vi "SR830 sweep tw.vi"(5 "Sweep":bool, 6 "Lock in parameters":T1={"Phase (deg)"=82.0, "TC"=7, "TC Multiplier"=5.0} {"TC Multiplier" min=0.0 max=10.0 step=1.0 format="%.2f"; "TC" items=["10 µs", "30 µs", "100 µs", "300 µs", "1 ms", "3 ms", "10 ms", "30 ms", "100 ms", "300 ms", "1 s", "3 s", "10 s", "30 s", "100 s", "300 s", "1 ks", "3 ks", "10 ks", "30 ks"]; "Phase (deg)" format="%.3f"}, 7 "Sweep frequency":T2={"Start Freq. (Hz)"=1040.0, "Stop Freq. (Hz)"=1200.0, "# of Steps"=100} {"Stop Freq. (Hz)" min=0.0 max=3000.0 step=0.001 format="%.3f"; "Start Freq. (Hz)" min=0.0 max=3000.0 step=0.001 format="%.3f"}, 8 "Lock-in GPIB address":string="0:9", 9 "SRS DS345 GPIB address":string="0:19") -> (0 "Fitting status":errorcluster[](array[cluster]), 1 "Best Fit Coefficients":dbl[][](array[numeric]) format="%#_6p", 2 "Sweep fit data":dbl[][](array[numeric]) format="%#_6p", 3 "Sweep data":dbl[][](array[numeric]) format="%#_6p")   [LabVIEW 2015]
uses:
  <vilib>/Analysis/1siggen.llb/Ramp Pattern by Samples.vi
  <vilib>/Analysis/baseanly.llb/Mean (DBL).vi
  <vilib>/gmath/NumericalOptimization/Nonlinear Curve Fit LM formula string.vi
  <vilib>/gmath/NI_Gmath.lvlib
  <vilib>/Analysis/NI_AALBase.lvlib
panel:
  out "Sweep Fit Chart":dbl[][](graph)
  out "Sweep Chart":cluster{"[0]":dbl, "[1]":dbl}(graph)
  in  "Lock-in GPIB address  (Fake)":string="1:8"
  # "width              center freq.        phase            amplitude        linear bkgd         cont bkgd\n        (Hz)                    (Hz)                (deg.)                (A)                   (A)                     (A)"
  # "X"
  # "Y"
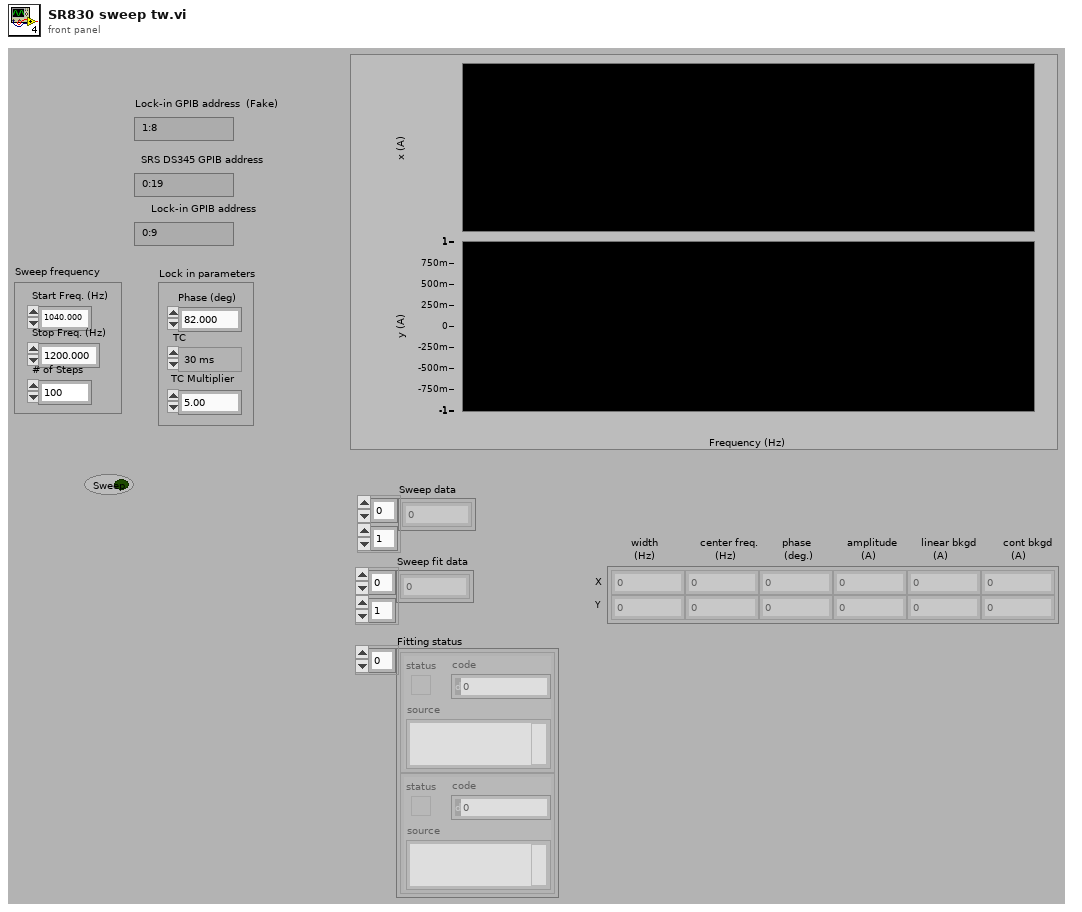
[diagram p1: front panel]
types:
  T1 = cluster{"Phase (deg)":dbl, "TC":i32, "TC Multiplier":dbl}
  T2 = cluster{"Start Freq. (Hz)":dbl, "Stop Freq. (Hz)":dbl, "# of Steps":u16}
  T3 = cluster{"Lock-in GPIB address  (Fake)":string, "Lock-in GPIB address  ":string, "SRS DS345 GPIB address":string}
  T4 = cluster{"model":string, "Parameters":string[], "x":string}
  T5 = cluster{"[0]":dbl, "[1]":dbl, "[2]":dbl, "[3]":dbl, "[4]":dbl, "[5]":dbl, "[6]":dbl, "[7]":dbl, "[8]":dbl}
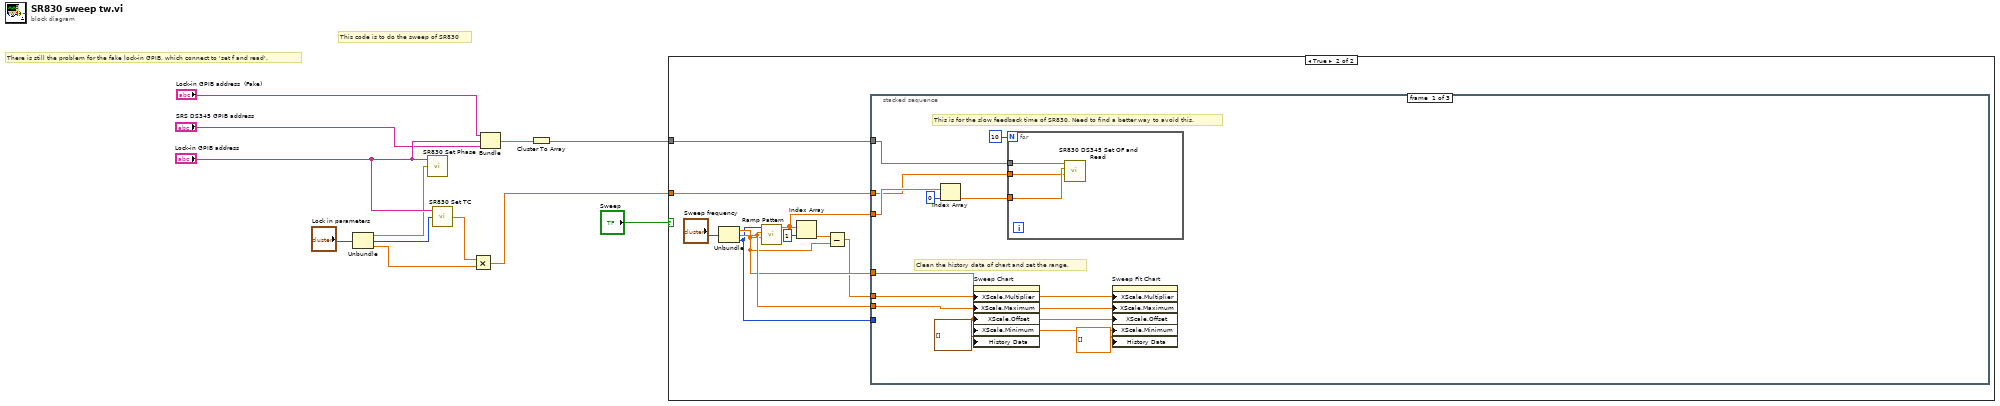
[diagram p0: block diagram]
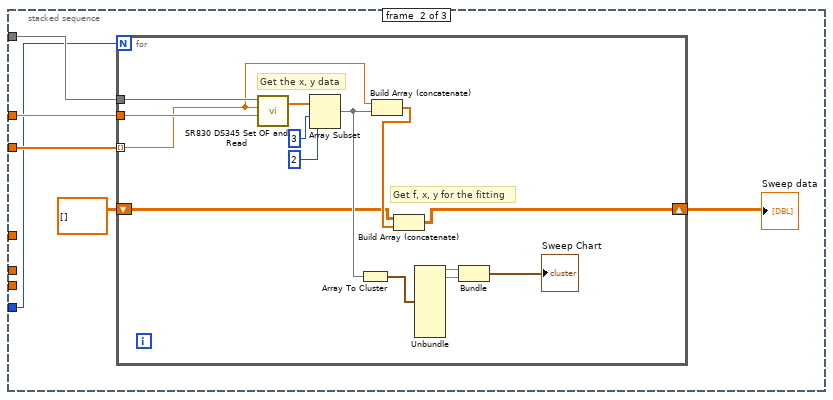
[diagram p3: hidden frame]
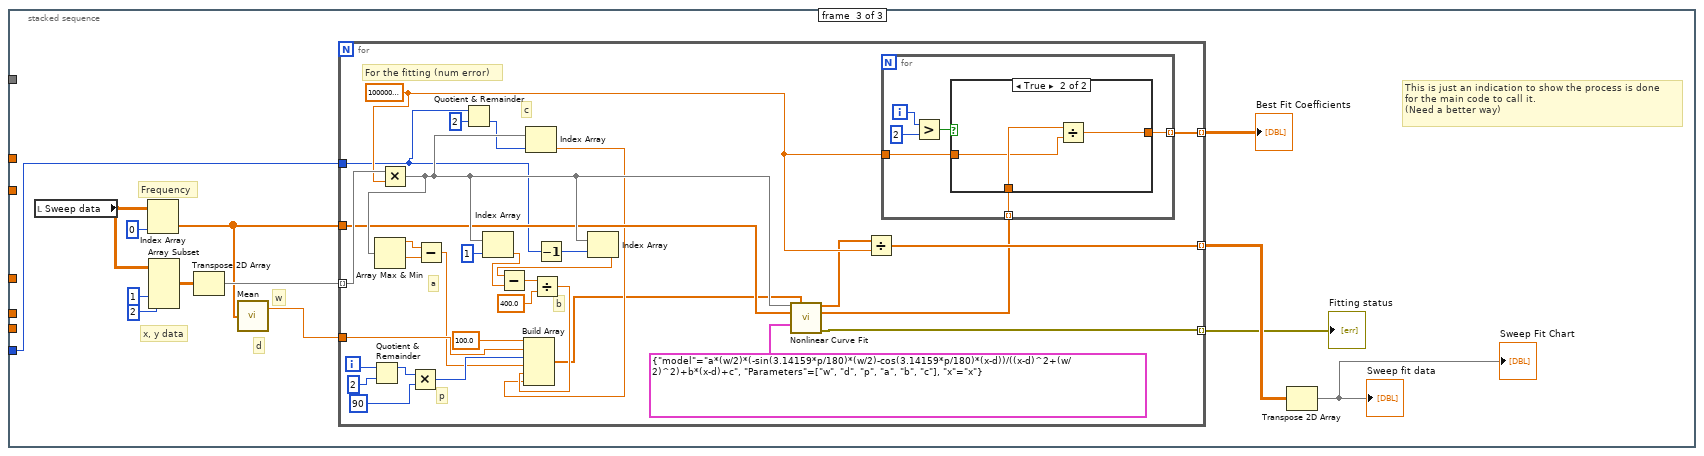
[diagram p4: hidden frame]
diagram:
  # "This code is to do the sweep of SR830"
  # "There is still the problem for the fake lock-in GPIB, which connect to 'set f and read'."
  n1 = Unbundle("Lock in parameters") -> ("Phase (deg)"=w4:dbl, "TC"=w3:i32, "TC Multiplier"=w2:dbl)
  n2 = call "SR830 Set Phase.vi"("Phase (deg)"=w4, "GPIB address"="Lock-in GPIB address") -> ()  [unwired: 2 in, 2 out]
  n3 = call "SR830 Set TC.vi"("time constant\n(10 µs : 0)"=w3, "GPIB address"="Lock-in GPIB address") -> ("tc (sec)"=w7:dbl)  [unwired: 1 in, 2 out]
  n4 = Multiply(x=w7, y=w2) -> (x*y=w6:dbl)
  n5 = Bundle("Lock-in GPIB address  (Fake)"="Lock-in GPIB address  (Fake)", "Lock-in GPIB address"="Lock-in GPIB address", "SRS DS345 GPIB address"="SRS DS345 GPIB address") -> (w9:T3)  [unwired: 1 out]
  n6 = Cluster To Array(cluster=w9) -> (array=w8:string[])
  n7 = case shown="True" "Sweep" {
    tunnel: w8 -> [_ w22]
    tunnel: w6 -> [_ w13]
    frame False {
    }
    frame True {
      n8 = Unbundle("Sweep frequency") -> ("Start Freq. (Hz)"=w17:dbl, "Stop Freq. (Hz)"=w20:dbl, "# of Steps"=w15:u16)
      n9 = call-poly <vilib>:"Ramp Pattern.vi"("start"=w17, "end"=w20, "samples"=w15) -> ("Ramp Pattern"=w14:dbl[])  [unwired: 7 in, 1 out]
      n10 = Index Array(array=w14, index=1) -> (element=w18:dbl)
      n11 = Subtract(x=w18, y=w17) -> (x-y=w16:dbl)
      n12 = stacked-sequence {
        tunnel: w22 -> [w30 w42 _]
        tunnel: w17 -> [w24 _ _]
        tunnel: w20 -> [w25 _ _]
        tunnel: w16 -> [w26 _ _]
        tunnel: w15 -> [_ w38 w58]
        tunnel: w14 -> [w33 w40 _]
        tunnel: w13 -> [w28 w41 _]
        frame #0 {
          # "This is for the slow feedback time of SR830. Need to find a better way to avoid this."
          # "Clean the history data of chart and set the range."
          n13 = Index Array(array=w33, index=0) -> (element=w29:dbl)
          n14 = property on="Sweep Chart" class="WFChart (strict)"("XScale.Multiplier"=w26, "XScale.Maximum"=w25, "XScale.Offset"=w24, "XScale.Minimum"=w24, "History Data"=cluster{"[0]":dbl, "[1]":dbl}[] []) -> ()  [unwired: 2 in, 2 out]
          n15 = for {
            N: 10 -> [_]
            tunnel: w30 -> [w36]
            tunnel: w29 -> [w35]
            tunnel: w28 -> [w34]
            n16 = call "SR830 DS345 Set OF and Read.vi"("Wait Time (sec)"=w34, "Oscillator Frequency (Hz)"=w35, "GPIB addresses"=w36) -> ()  [unwired: 1 in, 2 out]
          }
          n17 = property on="Sweep Fit Chart" class="WFChart (strict)"("XScale.Multiplier"=w26, "XScale.Maximum"=w25, "XScale.Offset"=w24, "XScale.Minimum"=w24, "History Data"=dbl[][] []) -> ()  [unwired: 2 in, 2 out]
        }
        frame #1 {
          n18 = for {
            N: w38 -> [_]
            tunnel: w42 -> [w56]
            tunnel: w40 -> [w47] mode=indexing
            tunnel: w41 -> [w55]
            shift-right: [w50] -> w37
            shift-left: dbl[][] [] -> [w46]
            # "Get f, x, y for the fitting"
            # "Get the x, y data"
            n19 = call "SR830 DS345 Set OF and Read.vi"("Wait Time (sec)"=w55, "Oscillator Frequency (Hz)"=w47, "GPIB addresses"=w56) -> ("f,x1,y1,x2,y2,aux11,aux12"=w54:dbl[])  [unwired: 1 in, 1 out]
            n20 = Array Subset(array=w54, index=3, length=2) -> (w48:dbl[])
            n21 = Array To Cluster(array=w48) -> (cluster=w51:T5)
            n22 = Build Array (concatenate)(w47, w48) -> (w49:dbl[])
            n23 = Build Array (concatenate)(w46, w49) -> (w50:dbl[][])
            n24 = Unbundle(w51) -> ("[0]"=w45:dbl, "[1]"=w44:dbl)  [unwired: 7 out]
            n25 = Bundle("[0]"=w45, "[1]"=w44) -> (→"Sweep Chart":cluster{"[0]":dbl, "[1]":dbl})  [unwired: 1 out]
          }
          "Sweep data" <- w37
        }
        frame #2 {
          # "This is just an indication to show the process is done\nfor the main code to call it. \n(Need a better way)"
          # "d"
          # "w"
          # "x, y data"
          # "Frequency"
          n26 = local read "Sweep data"() -> (w68:dbl[][])
          n27 = Index Array(array=w68, index (col)=0 ("disabled index (col)")) -> (element=w63:dbl[])  [unwired: 1 in]
          n28 = Array Subset(array=w68, index (col)=1 ("index"), length (col)=2 ("length")) -> (w65:dbl[][])  [unwired: 2 in]
          n29 = Transpose 2D Array(2D array=w65) -> (transposed array=w64:dbl[][])
          n30 = call-poly <vilib>:"Mean.vi"("X"=w63) -> ("mean"=w59:dbl)  [unwired: 1 out]
          n31 = for {
            tunnel: w63 -> [w85]
            tunnel: w64 -> [w97] mode=indexing
            tunnel: [w89] -> w62 mode=indexing
            tunnel: [w87] -> w61 mode=indexing
            tunnel: [w81] -> w60 mode=indexing
            tunnel: w59 -> [w79]
            tunnel: w58 -> [w72]
            i -> [w101]
            w88 = 1000000000000.0 ("y")
            # "b"
            # "c"
            # "a"
            # "p"
            # "For the fitting (num error)"
            n32 = Quotient & Remainder(x=w101, y=2) -> (x-y*floor(x/y)=w99:i32)  [unwired: 1 out]
            n33 = Multiply(x=w97, y=w88) -> (x*y=w86:dbl[])
            n34 = Array Max & Min(array=w86) -> (max value=w96:dbl, min value=w95:dbl)  [unwired: 2 out]
            n35 = Multiply(x=w99, y=90) -> (x*y=w78:i32)
            n36 = Subtract(x=w96, y=w95) -> (x-y=w77:dbl)
            n37 = Quotient & Remainder(x=w72, y=2 ("index")) -> (floor(x/y)=w71:i32)  [unwired: 1 out]
            n38 = Index Array(array=w86, index=1) -> (element=w92:dbl)
            n39 = Index Array(array=w86, index=w71) -> (element=w75:dbl)
            n40 = Decrement(x=w72) -> (x-1=w73:u16)
            n41 = Index Array(array=w86, index=w73) -> (element=w93:dbl)
            n42 = Subtract(x=w93, y=w92) -> (x-y=w91:dbl)
            n43 = Divide(x=w91, y=400.0) -> (x/y=w76:dbl)
            n44 = Build Array(100.0, w79, w78, w77, w76, w75) -> (w74:dbl[])
            n45 = call-poly <vilib>:"Nonlinear Curve Fit.vi"("Y"=w86, "initial parameters"=w74, "X"=w85, "model description"=T4 {"model"="a*(w/2)*(-sin(3.14159*p/180)*(w/2)-cos(3.14159*p/180)*(x-d))/((x-d)^2+(w/2)^2)+b*(x-d)+c", "Parameters"=["w", "d", "p", "a", "b", "c"], "x"="x"}) -> ("best nonlinear fit"=w83:dbl[], "best fit parameters"=w84:dbl[], "error out"=w81:errorcluster)  [unwired: 3 in, 6 out]
            n46 = Divide(x=w83, y=w88) -> (x/y=w89:dbl[])
            n47 = for {
              tunnel: w84 -> [w104] mode=indexing
              tunnel: w88 -> [w103]
              tunnel: [w102] -> w87 mode=indexing
              i -> [w107]
              n48 = Greater?(x=w107, y=2) -> (0:w105:bool)
              n49 = case shown="True" w105 {
                tunnel: w104 -> [w108 w111]
                tunnel: w103 -> [_ w110]
                tunnel: [w108 w109] -> w102
                frame False {
                }
                frame True {
                  n50 = Divide(x=w111, y=w110) -> (x/y=w109:dbl)
                }
              }
            }
          }
          "Best Fit Coefficients" <- w61
          "Fitting status" <- w60
          n51 = Transpose 2D Array(2D array=w62) -> (transposed array=→"Sweep fit data" →"Sweep Fit Chart":dbl[][])
        }
      }
    }
  }
